vi "ALARM Message Loop.vi"(8 "error in (no error)":errorcluster) -> (0 "error out":errorcluster)   [LabVIEW 2020, in "QCT ALARM.lvlib"]
doc: "Message loop for handling messages pertaining to the acquisition of data from the hardware."
uses:
  QCT ALARM.lvlib
  support/PCT FGV CMD.ctl
  Acquisition State.ctl
  ALARM Configuration.ctl
  support/Message Queue/Message Cluster.ctl
  support/Message Queue/Enqueue Message (Single).vi
  <vilib>/Utility/error.llb/Error Cluster From Error Code.vi
  <vilib>/ErrorRing/Error Ring.xnode
  support/Message Queue/Message Queue.lvlib
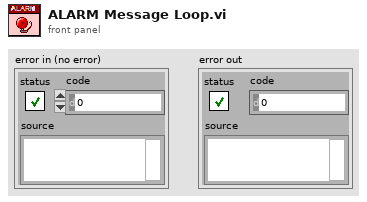
[diagram p1: front panel]
types:
  T1 = typedef "PCT FGV CMD.ctl" = enum16{"INIT", "GET", "SET"}
  T2 = typedef "PCT Data REFs.ctl" = cluster{"PLC AI Notifier":refnum<notifier>, "PS Data Queue":refnum<queue>, "BTN Queue":refnum<queue>, "PLC DI notifier":refnum<notifier>, "Timer notifier":refnum<notifier>, "DMM PS":refnum<notifier>, "DMM Gages":refnum<notifier>, "XYZ notifier":refnum<notifier>, "Test Notifier":refnum<notifier>, "Scanner notifier":refnum<notifier>, "OPC Notifier":refnum<notifier>, "HIDEN queue":refnum<queue>}
  T3 = typedef "Message Queue.lvlib/All Message Queues.ctl" = cluster{"UI":refnum<queue>, "Logging":refnum<queue>, "LOG":refnum<queue>, "ALARM":refnum<queue>, "Test":refnum<queue>, "Answer":refnum<queue>, "PLC":refnum<queue>, "DB":refnum<queue>, "Report":refnum<queue>, "OPC":refnum<queue>, "Procedure":refnum<queue>, "PalmSens":refnum<queue>, "SYS 7000 Reader":refnum<queue>, "SWITCH":refnum<queue>, "MOTOR":refnum<queue>, "MOTION":refnum<queue>, "HIDEN":refnum<queue>, "VALVE":refnum<queue>, "MFC":refnum<queue>, "PUMP IN":refnum<queue>, "PUMP OUT":refnum<queue>}
  T4 = typedef "QCT ALARM.lvlib/ALARM Configuration.ctl" = cluster{"LOG REF":refnum<vi>, "Writer Queue":refnum<queue>, "Log Path":path, "UPS standby":bool, "status code":i32, "SP":dbl[], "Over Sens Status":dbl[]}
  T5 = typedef "QCT ALARM.lvlib/Acquisition State.ctl" = enum16{"Idle", "Initialized"}
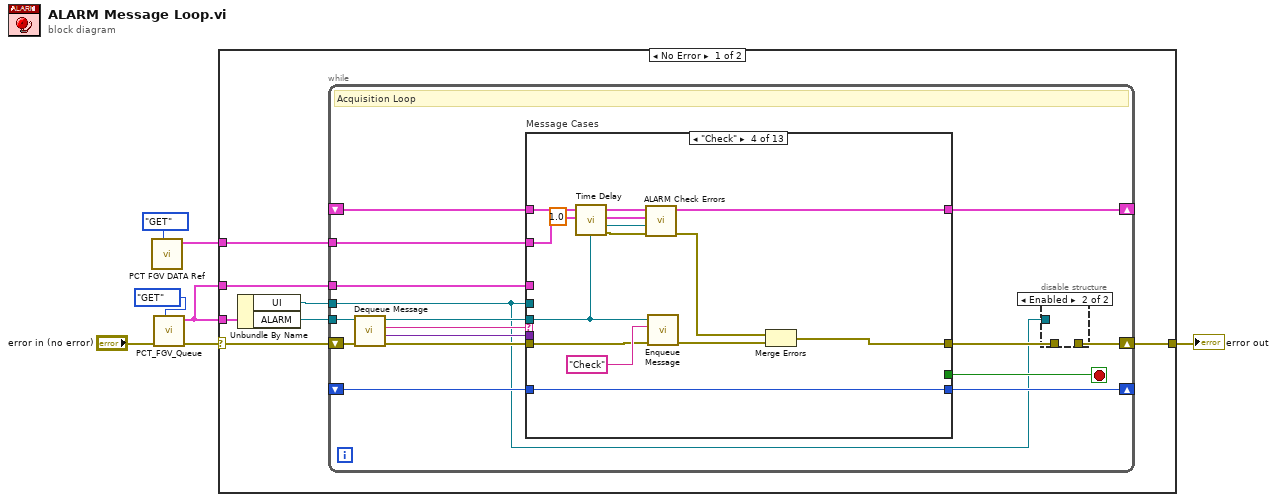
[diagram p0: block diagram]
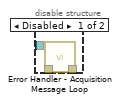
[diagram p2: hidden frame]
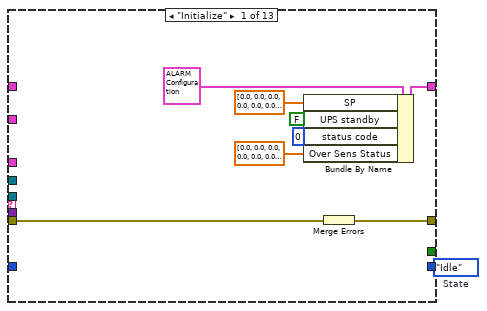
[diagram p3: hidden frame]
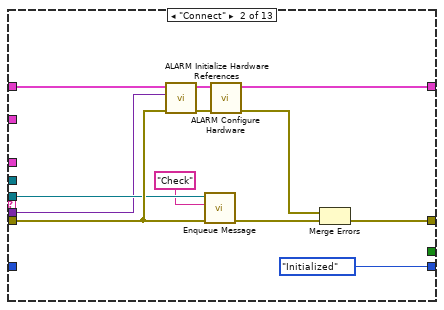
[diagram p4: hidden frame]
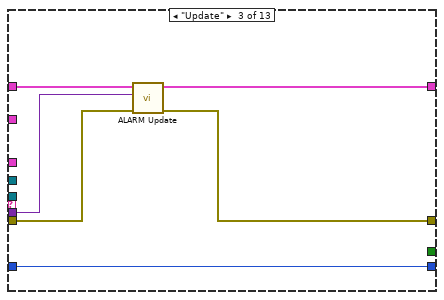
[diagram p5: hidden frame]
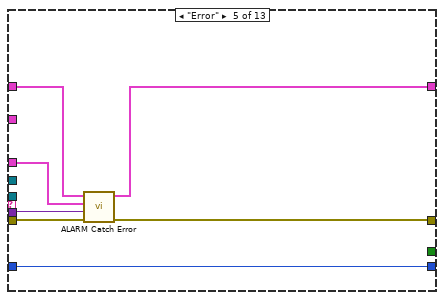
[diagram p6: hidden frame]
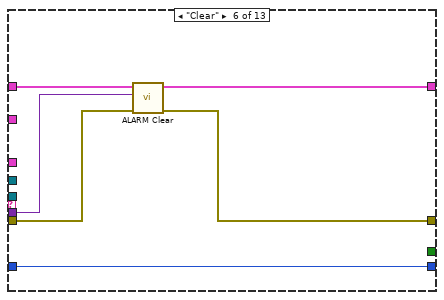
[diagram p7: hidden frame]
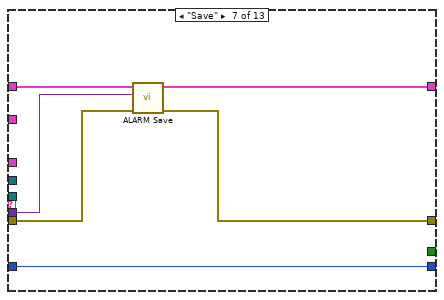
[diagram p8: hidden frame]
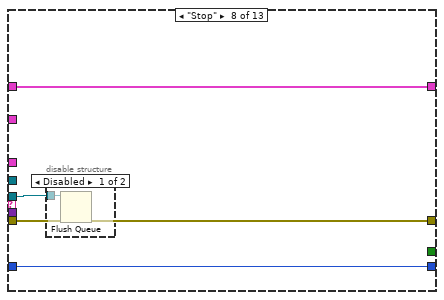
[diagram p9: hidden frame]
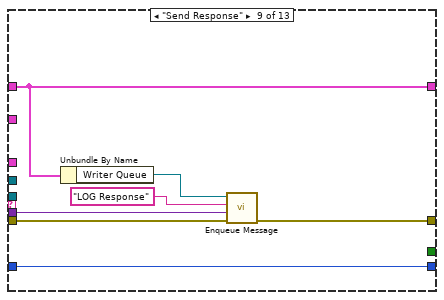
[diagram p11: hidden frame]
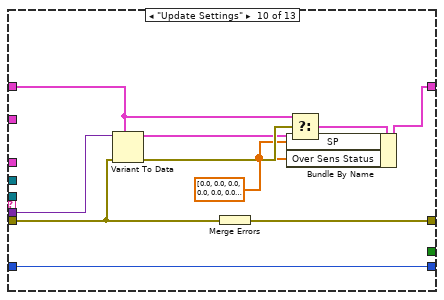
[diagram p12: hidden frame]
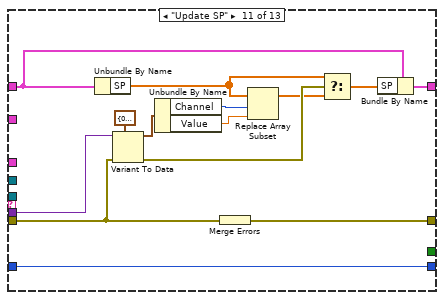
[diagram p13: hidden frame]
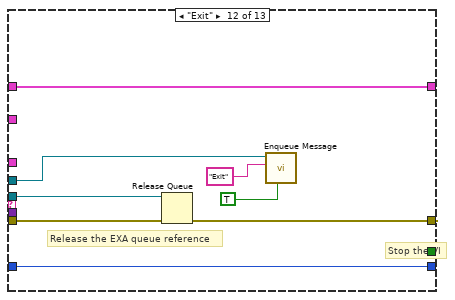
[diagram p14: hidden frame]
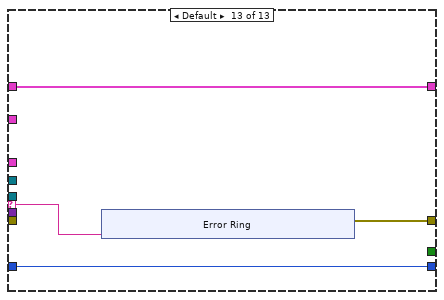
[diagram p15: hidden frame]
diagram:
  n1 = call "PCT FGV DATA Ref.vi"("CMD"=PCT_FGV_CMD."GET") -> ("Data REF"=w1:T2)  [unwired: 9 in, 1 out]
  n2 = call "PCT_FGV_Queue.vi"("CMD"=PCT_FGV_CMD."GET", "error in (no error)"="error in (no error)") -> ("error out"=w4:errorcluster, "Message Queues out"=w3:T3)  [unwired: 8 in]
  n3 = case shown="No Error" w4 {
    selector: w4 -> [w11 w149]
    tunnel: w3 -> [w14 _]
    tunnel: [w12 w149] -> w7
    tunnel: w3 -> [w9 _]
    tunnel: w1 -> [w8 _]
    frame No Error {
      n4 = Unbundle By Name(w14) -> ("UI"=w10:refnum<queue>, "ALARM"=w13:refnum<queue>)
      n5 = while {
        tunnel: w13 -> [w23]
        shift-right: [w29] -> _
        shift-left: _ -> [w30]
        shift-right: [w20] -> w12
        shift-left: w11 -> [w27]
        tunnel: w10 -> [w17]
        shift-right: [w21] -> _
        shift-left: _ -> [w22]
        tunnel: w9 -> [w16]
        tunnel: w8 -> [w15]
        stop <- w28 stop-if-true
        # "Acquisition Loop"
        n6 = call "Dequeue Message.vi"("error in (no error)"=w27, "Message Queue"=w23) -> ("error out"=w26:errorcluster, "Message Data"=w24:variant, "Message"=w25:string, "dup Message Queue"=w18:refnum<queue>)  [unwired: 6 in]
        n7 = case "Message Cases" shown="\"Check\"" w25 {
          selector: w25 -> [_ _ _ _ _ _ _ _ _ _ _ _ w138]
          tunnel: w18 -> [_ w51 _ w63 _ _ _ w92 _ _ _ w129 _]
          tunnel: w26 -> [w41 w52 w56 w66 w77 w81 w87 w95 w101 w107 w124 w133 _]
          tunnel: [w42 w54 w55 w65 w78 w80 w86 w95 w100 w113 w127 w136 w139] -> w19
          tunnel: w30 -> [_ w53 w57 w71 w74 w82 w88 w94 w98 w109 w116 w135 w141]
          tunnel: [w38 w50 w58 w70 w73 w83 w89 w94 w98 w105 w115 w135 w141] -> w29
          tunnel: [_ _ _ _ _ _ _ _ _ _ _ TRUE _] -> w28
          tunnel: w24 -> [_ w48 w59 _ w76 w84 w90 _ w99 w112 w126 _ _]
          tunnel: w17 -> [_ _ _ _ _ _ _ _ _ _ _ w134 _]
          tunnel: w22 -> [_ _ w60 w72 w79 w85 w91 w93 w102 w106 w123 w128 w140]
          tunnel: [w40 Acquisition_State."Initialized" ("Acquisition State") w60 w72 w79 w85 w91 w93 w102 w106 w123 w128 w140] -> w21
          tunnel: w16 -> [_ _ _ _ w75 _ _ _ _ _ _ _ _]
          tunnel: w15 -> [_ _ _ w68 _ _ _ _ _ _ _ _ _]
          frame "Initialize" {
            w40 = Acquisition_State."Idle"  # State
            # "Initialize  - Initialize is currently a no-op.  The hardware initialization takes place in the 'Start' message."
            n8 = Bundle By Name(cluster=T4 {"LOG REF"=refnum, "Writer Queue"=refnum, "Log Path"=path "", "UPS standby"=FALSE, "status code"=5001, "SP"=[], "Over Sens Status"=[]} ("Data Cluster"), "SP"=dbl[] [0.0, 0.0, 0.0, 0.0, 0.0, 0.0, 0.0, 0.0, 0.0, 0.0], "UPS standby"=FALSE, "status code"=0, "Over Sens Status"=dbl[] [0.0, 0.0, 0.0, 0.0, 0.0, 0.0, 0.0, 0.0, 0.0, 0.0, 0.0, 0.0, 0.0, 0.0, 0.0, 0.0, 0.0, 0.0, 0.0, 0.0, 0.0, 0.0, 0.0, 0.0, 0.0, 0.0, 0.0, 0.0, 0.0, 0.0, 0.0, 0.0, 0.0, 0.0, 0.0, 0.0, 0.0, 0.0, 0.0, 0.0, 0.0, 0.0, 0.0, 0.0, 0.0, 0.0, 0.0, 0.0, 0.0, 0.0, 0.0, 0.0, 0.0, 0.0, 0.0, 0.0, 0.0, 0.0, 0.0, 0.0, 0.0, 0.0, 0.0, 0.0, 0.0, 0.0, 0.0, 0.0, 0.0, 0.0, 0.0, 0.0, 0.0, 0.0, 0.0, 0.0, 0.0, 0.0, 0.0, 0.0] ("SP")) -> (w38:T4)
            n9 = Merge Errors(w41) -> (w42:errorcluster)
          }
          frame "Connect" {
            # "Start - Configure and start the acquisition."
            n10 = call "ALARM Initialize Hardware References.vi"("error in (no error)"=w52, "Message Data"=w48, "Hardware Resources in"=w53) -> ("error out"=w47:errorcluster, "Hardware Resources out"=w45:T4)  [unwired: 7 in]
            n11 = call-poly "Enqueue Message.vi"("error in (no error)"=w52, "Message"="Check", "Message Queue"=w51) -> ("error out"=w44:errorcluster)  [unwired: 7 in, 1 out]
            n12 = call "ALARM Configure Hardware.vi"("error in (no error)"=w47, "Hardware Resources in"=w45) -> ("error out"=w46:errorcluster, "Hardware Resources out"=w50:T4)  [unwired: 8 in]
            n13 = Merge Errors(w46, w44) -> (w54:errorcluster)
          }
          frame "Update" {
            # "Start - Configure and start the acquisition."
            n14 = call "ALARM Update.vi"("error in (no error)"=w56, "Message Data"=w59, "Data Cluster"=w57) -> ("error out"=w55:errorcluster, "Data Cluster out"=w58:T4)  [unwired: 7 in]
          }
          frame "Check" {
            # "Start - Configure and start the acquisition."
            n15 = call "Time Delay"("Delay Time (s)"=1.0) -> ("error out"=w62:errorcluster)  [unwired: 10 in]
            n16 = call "ALARM Check Errors.vi"("error in (no error)"=w62, "ALARM Q"=w63, "Data REF"=w68, "Data Cluster"=w71) -> ("error out"=w69:errorcluster, "Data Cluster out"=w70:T4)  [unwired: 6 in]
            n17 = call-poly "Enqueue Message.vi"("error in (no error)"=w66, "Message"="Check", "Message Queue"=w63) -> ("error out"=w64:errorcluster)  [unwired: 7 in, 1 out]
            n18 = Merge Errors(w69, w64) -> (w65:errorcluster)
          }
          frame "Error" {
            n19 = call "ALARM Catch Error.vi"("error in (no error)"=w77, "Data"=w76, "Message Queues out"=w75, "Hardware Resources in"=w74) -> ("error out"=w78:errorcluster, "Hardware Resources out"=w73:T4)  [unwired: 6 in]
          }
          frame "Clear" {
            # "Start - Configure and start the acquisition."
            n20 = call "ALARM Clear.vi"("error in (no error)"=w81, "Message Data"=w84, "Data Cluster"=w82) -> ("error out"=w80:errorcluster, "Data Cluster out"=w83:T4)  [unwired: 7 in]
          }
          frame "Save" {
            # "Start - Configure and start the acquisition."
            n21 = call "ALARM Save.vi"("error in (no error)"=w87, "Message Data"=w90, "Data Cluster"=w88) -> ("error out"=w86:errorcluster, "Data Cluster out"=w89:T4)  [unwired: 7 in]
          }
          frame "Stop" {
            n22 = disable-structure shown="Disabled" {
              disable-tunnel: w92 -> [w96 _]
              frame Disabled {
                n23 = Flush Queue(queue=w96) -> ()  [unwired: 1 in, 3 out]
              }
              frame Enabled {
              }
            }
          }
          frame "Send Response" {
            # "Acquire - Acquire data from the hardware. Since this is a continuous acquisition, this message will always message itself to run again."
            n24 = Unbundle By Name(w98) -> ("Writer Queue"=w97:refnum<queue>)
            n25 = call-poly "Enqueue Message.vi"("error in (no error)"=w101, "Message Data"=w99, "Message"="LOG Response", "Message Queue"=w97) -> ("error out"=w100:errorcluster)  [unwired: 6 in, 1 out]
          }
          frame "Update Settings" {
            w104 = dbl[] [0.0, 0.0, 0.0, 0.0, 0.0, 0.0, 0.0, 0.0, 0.0, 0.0] ("SP")
            # "New settings are available, update the current ones stored in the shift register with the settings sent as part of the message"
            n26 = Variant To Data(error in=w107, type=w109, Variant=w112) -> (data=w110:T4, error out=w111:errorcluster)
            n27 = Merge Errors(w107) -> (w113:errorcluster)
            n28 = Select(t=w109, s=w111, f=w110) -> (s? t:f=w108:T4)
            n29 = Bundle By Name(cluster=w108, "SP"=w104, "Over Sens Status"=w104) -> (w105:T4)
          }
          frame "Update SP" {
            # "New settings are available, update the current ones stored in the shift register with the settings sent as part of the message"
            n30 = Unbundle By Name(w116) -> ("SP"=w117:dbl[])
            n31 = Variant To Data(error in=w124, type=cluster{"Value":dbl, "Channel":i32} {"Value"=0.0, "Channel"=0} ("Data"), Variant=w126) -> (data=w121:cluster{"Value":dbl, "Channel":i32}, error out=w125:errorcluster)
            n32 = Unbundle By Name(w121) -> ("Channel"=w120:i32, "Value"=w119:dbl)
            n33 = Merge Errors(w124) -> (w127:errorcluster)
            n34 = Replace Array Subset(array=w117, new element=w119, index=w120) -> (w118:dbl[])
            n35 = Select(t=w117, s=w125, f=w118) -> (s? t:f=w114:dbl[])
            n36 = Bundle By Name(cluster=w116, "SP"=w114) -> (w115:T4)
          }
          frame "Exit" {
            # "Release the EXA queue reference"
            # "Stop the VI"
            # "Exit - Send the Exit message to the UI Message Handler."
            n37 = Release Queue(queue=w129, error in (no error)=w133) -> (error out=w130:errorcluster)  [unwired: 1 in, 2 out]
            n38 = call-poly "Enqueue Message.vi"("Priority Message? (F)"=TRUE, "Message"="Exit", "Message Queue"=w134) -> ()  [unwired: 7 in, 2 out]
            n39 = Merge Errors(w130) -> (w136:errorcluster)
          }
          frame Default {
            # "'Default' case only runs if there is a message that isn't defined in any of the other cases.  Output a programming error."
            n40 = xnode "Error Ring"("parameter 0"=w138) -> ("error out"=w139:errorcluster)
          }
        }
        n41 = disable-structure shown="Enabled" {
          disable-tunnel: [w33 _] -> w20
          disable-tunnel: w19 -> [w32 _]
          disable-tunnel: w17 -> [w31 _]
          frame Disabled {
            n42 = call "Error Handler - Acquisition Message Loop.vi"("error in (no error)"=w32, "Message Queue"=w31) -> ("dup error in"=w33:errorcluster)  [unwired: 8 in, 1 out]
          }
          frame Enabled {
          }
        }
      }
    }
    frame Error {
    }
  }
  "error out" <- w7
